vi "Disable All Steps.vi"(8 "error in (no error)":errorcluster, 11 "Steps in":refnum<class "Steps.lvclass">) -> (0 "error out":errorcluster, 3 "Steps out":refnum<class "Steps.lvclass">)   [LabVIEW 2015, in "Steps.lvclass"]
doc: "<b> </b> <b> </b>\n©2016 Q Software Innovations, LLC (QSI)\nwritten by Quentin Alldredge\nproduced in LabVIEW 2015\n\nsupport@qsoftwareinnovations.com\nwww.qsoftwareinnovations.com\n\nAll rights reserved.\n\nRedistribution and use in source and binary forms, with or without modification, are permitted provided that the following conditions are met:\n\n * Redistributions of source code must retain the above copyright notice, this list of conditions and the following disclaimer.\n * Redistributions in binary form must reproduce the above copyright notice, this list of conditions and the following disclaimer in the documentation and/or other materials provided with the distribution.\n * Neither the name of Q Software Innovations, LLC. nor the names of its contributors may be used to endorse or promote products derived from this software without specific prior written permission.\n\nTHIS SOFTWARE IS PROVIDED BY THE COPYRIGHT HOLDERS AND CONTRIBUTORS \"AS IS\" AND ANY EXPRESS OR IMPLIED WARRANTIES, INCLUDING, BUT NOT LIMITED TO, THE IMPLIED WARRANTIES OF MERCHANTABILITY AND FITNESS FOR A PARTICULAR PURPOSE ARE DISCLAIMED. IN NO EVENT SHALL THE COPYRIGHT OWNER OR CONTRIBUTORS BE LIABLE FOR ANY DIRECT, INDIRECT, INCIDENTAL, SPECIAL, EXEMPLARY, OR CONSEQUENTIAL DAMAGES (INCLUDING, BUT NOT LIMITED TO, PROCUREMENT OF SUBSTITUTE GOODS OR SERVICES; LOSS OF USE, DATA, OR PROFITS; OR BUSINESS INTERRUPTION) HOWEVER CAUSED AND ON ANY THEORY OF LIABILITY, WHETHER IN CONTRACT, STRICT LIABILITY, OR TORT (INCLUDING NEGLIGENCE OR OTHERWISE) ARISING IN ANY WAY OUT OF THE USE OF THIS SOFTWARE, EVEN IF ADVISED OF THE POSSIBILITY OF SUCH DAMAGE."
uses:
  Steps.lvclass
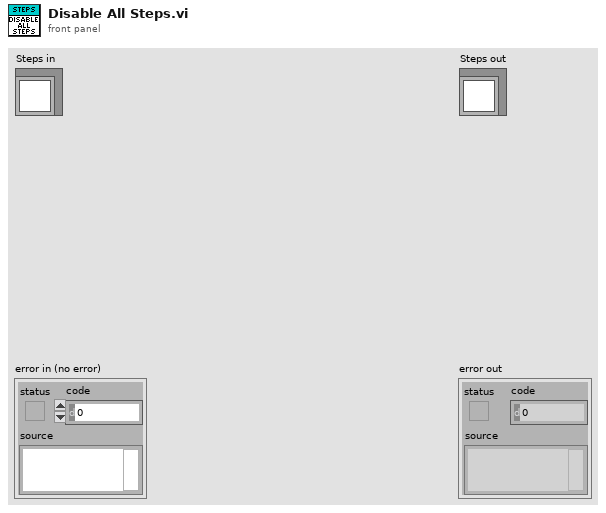
[diagram p1: front panel]
types:
  T1 = enum32{"Page Enabled", "Page Disabled", "Page Disabled & Grayed"}
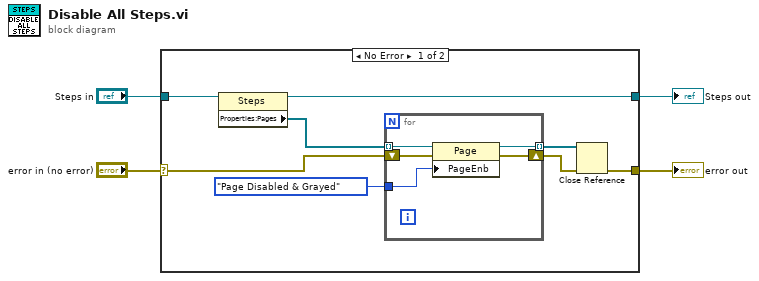
[diagram p0: block diagram]
diagram:
  n1 = case shown="No Error" "error in (no error)" {
    selector: "error in (no error)" -> [w9 w19]
    tunnel: [w5 w19] -> w3
    tunnel: [w11 w18] -> w1
    tunnel: "Steps in" -> [w12 w18]
    frame No Error {
      n2 = property class="Steps"(reference=w12) -> (reference out=w11:refnum<class "Steps.lvclass">, "Properties:Pages"=w10:refnum<vi>[])  [unwired: 1 in, 1 out]
      n3 = for {
        tunnel: w10 -> [w17] mode=indexing
        tunnel: T1."Page Disabled & Grayed" ("Page Enabled State") -> [w15]
        tunnel: [w14] -> w7 mode=indexing
        shift-right: [w13] -> w6
        shift-left: w9 -> [w16]
        n4 = property class="Page"(reference=w17, error in=w16, "PageEnb"=w15) -> (reference out=w14:refnum<vi>, error out=w13:errorcluster)
      }
      n5 = Close Reference(reference=w7, error in (no error)=w6) -> (error out=w5:errorcluster)
    }
    frame Error {
    }
  }
  "error out" <- w3
  "Steps out" <- w1
